vi "Load Robot Parameters.vi"(8 "error in (no error)":errorcluster, 11 "Stop on error":bool) -> (0 "error out":errorcluster)   [LabVIEW 2015]
uses:
  Robot Parameters.ctl
  Arm Mode TypeDef.ctl
  <vilib>/Utility/xml.llb/Read From XML File(string).vi
  Global Variables.vi
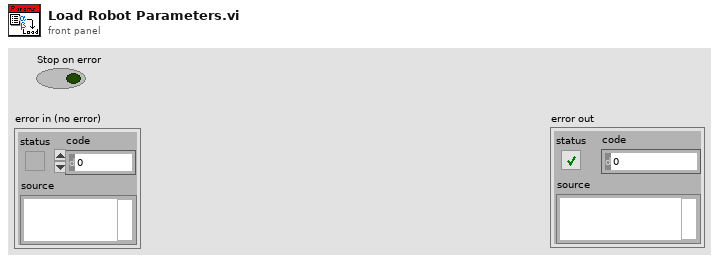
[diagram p1: front panel]
types:
  T1 = typedef "Robot Parameters.ctl" = cluster{"Robot Drive Parameters":cluster{"Teleop Drive Mode":enum16{"Split Axis Arcade", "Arcade Drive", "Tank Drive"}, "Drive PID Gains":cluster{"GRIP - Centering":cluster{"proportional gain (Kc)":dbl, "integral time (Ti, min)":dbl, "derivative time (Td, min)":dbl}, "Encoder":cluster{"proportional gain (Kc)":dbl, "integral time (Ti, min)":dbl, "derivative time (Td, min)":dbl}, "IMU - Spin":cluster{"proportional gain (Kc)":dbl, "integral time (Ti, min)":dbl, "derivative time (Td, min)":dbl}}, "Slew Rate (Units / Second)":dbl}, "Shooter Parameters":cluster{"Open Claw Delay":u32, "Shoot Delay":u32, "Pressure Threshold for shooting":dbl, "Arm Position Interlock Angle":dbl}, "Arm Parameters":cluster{"PID gains":cluster{"proportional gain (Kc)":dbl, "integral time (Ti, min)":dbl, "derivative time (Td, min)":dbl}, "Arm Max Angle":dbl, "Arm Min Angle":dbl, "Default Angle":dbl, "Shoot Batter Angle":dbl, "Shoot Close Angle":dbl, "Shoot Far Angle":dbl, "Human Player Load Angle":dbl, "Low Bar / Goal Angle":dbl, "Driver - Cross Defense Angle":dbl, "Arm Position Sensor Map":cluster{"Input Low (V)":dbl, "Input High (V)":dbl, "Output Low (Degree)":dbl, "Output High (Degree)":dbl}, "Arm Position Tolerance":dbl, "Disable Lock Modes":T2[]}, "Intake Parameters":cluster{"Suck In Speed":dbl, "Spit Out Speed":dbl}}
  T2 = typedef "Arm Mode TypeDef.ctl" = enum16{"Unknown", "Disabled", "Locked", "Shoot Batter", "Shoot Close", "Cross Defense", "Human Player Load", "Low Bar / Goal", "Manual"}
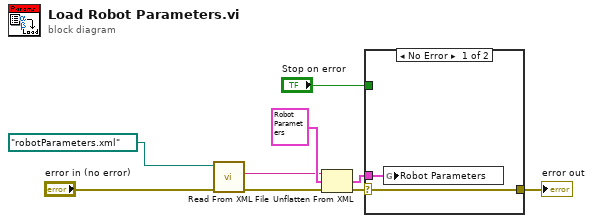
[diagram p0: block diagram]
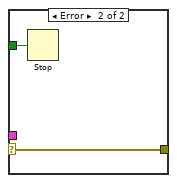
[diagram p2: hidden frame]
diagram:
  n1 = call-poly <vilib>:"Read From XML File.vi"("error in (no error)"="error in (no error)", "XML File Path"=path "/robotParameters.xml") -> ("error out"=w5:errorcluster, "XML Elements"=w6:string)  [unwired: 7 in, 1 out]
  n2 = Unflatten From XML(xml string=w6, type=T1 {"Robot Drive Parameters"={"Teleop Drive Mode"=enum."Split Axis Arcade", "Drive PID Gains"={"GRIP - Centering"={"proportional gain (Kc)"=1.0, "integral time (Ti, min)"=0.01, "derivative time (Td, min)"=0.0}, "Encoder"={"proportional gain (Kc)"=0.0, "integral time (Ti, min)"=0.0, "derivative time (Td, min)"=0.0}, "IMU - Spin"={"proportional gain (Kc)"=0.04000000000000001, "integral time (Ti, min)"=0.02, "derivative time (Td, min)"=0.0}}, "Slew Rate (Units / Second)"=0.0}, "Shooter Parameters"={"Open Claw Delay"=200, "Shoot Delay"=300, "Pressure Threshold for shooting"=75.0, "Arm Position Interlock Angle"=0.0}, "Arm Parameters"={"PID gains"={"proportional gain (Kc)"=1.0, "integral time (Ti, min)"=0.01, "derivative time (Td, min)"=0.0}, "Arm Max Angle"=180.0, "Arm Min Angle"=100.0, "Default Angle"=140.0, "Shoot Batter Angle"=140.0, "Shoot Close Angle"=140.0, "Shoot Far Angle"=140.0, "Human Player Load Angle"=140.0, "Low Bar / Goal Angle"=140.0, "Driver - Cross Defense Angle"=0.0, "Arm Position Sensor Map"={"Input Low (V)"=0.0, "Input High (V)"=0.0, "Output Low (Degree)"=0.0, "Output High (Degree)"=0.0}, "Arm Position Tolerance"=0.0, "Disable Lock Modes"=[enum."Manual"]}, "Intake Parameters"={"Suck In Speed"=0.0, "Spit Out Speed"=0.0}}, error in (no error)=w5) -> (value=w8:T1, error out=w7:errorcluster)
  n3 = case shown="No Error" w7 {
    selector: w7 -> [w10 w13]
    tunnel: w8 -> [w11 _]
    tunnel: [w10 w13] -> w2
    tunnel: "Stop on error" -> [_ w12]
    frame No Error {
      n4 = global write "Global Variables.vi" "Robot Parameters"(w11) -> ()
    }
    frame Error {
      n5 = Stop(stop? (T)=w12) -> ()
    }
  }
  "error out" <- w2
